vi "Transmisor SERIALvi.vi"() -> ()   [LabVIEW 2020]
uses:
  <vilib>/Instr/_visa.llb/VISA Configure Serial Port (Instr).vi
panel:
  in  "ConfigSerial":T1={"baud rate (9600)"=9600, "data bits (8)"=8, "parity (0:none)"=enum."None", "stop bits (10: 1 bit)"=10, "flow control (0:none)"=0, "VISA resource name"="", "error in (no error) 2"={"status"=FALSE, "code"=0, "source"=""}} {"flow control (0:none)" items=["None", "XON/XOFF", "RTS/CTS", "XON/XOFF & RTS/CTS", "DTR/DSR", "XON/XOFF & DTR/DSR"]; "stop bits (10: 1 bit)" items=["1.0"=10, "1.5"=15, "2.0"=20]; "data bits (8)" min=5 max=8 step=1}
  in  "Stop":bool
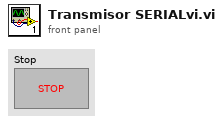
[diagram p1: front panel]
types:
  T1 = cluster{"baud rate (9600)":u32, "data bits (8)":u16, "parity (0:none)":enum16{"None", "Odd", "Even", "Mark", "Space"}, "stop bits (10: 1 bit)":u16, "flow control (0:none)":u16, "VISA resource name":refnum<visa-resource-name>, "error in (no error) 2":errorcluster}
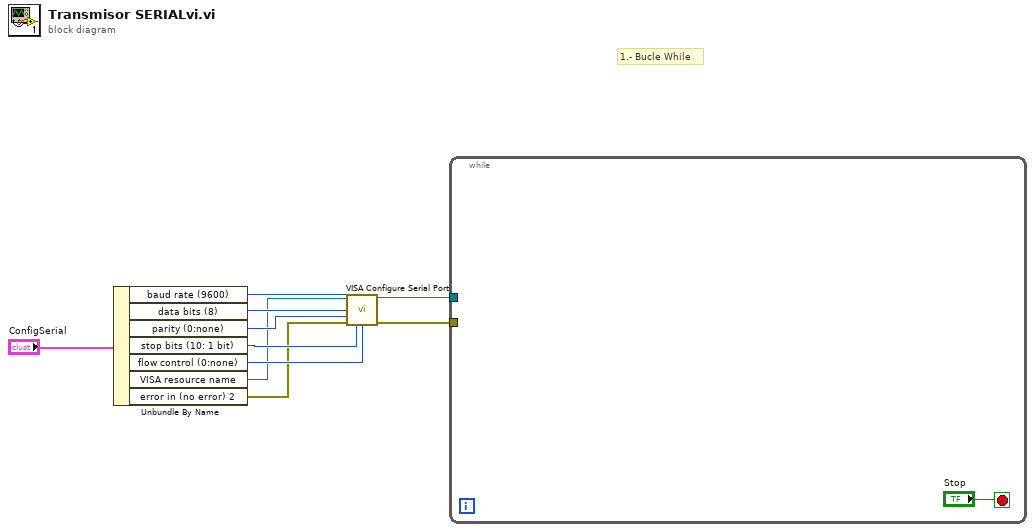
[diagram p0: block diagram]
diagram:
  # "1.- Bucle While"
  n1 = Unbundle By Name("ConfigSerial") -> ("baud rate (9600)"=w9:u32, "data bits (8)"=w8:u16, "parity (0:none)"=w7:enum16{"None", "Odd", "Even", "Mark", "Space"}, "stop bits (10: 1 bit)"=w6:u16, "flow control (0:none)"=w5:u16, "VISA resource name"=w4:refnum<visa-resource-name>, "error in (no error) 2"=w3:errorcluster)
  n2 = call-poly "VISA Configure Serial Port"("VISA resource name"=w4, "baud rate (9600)"=w9, "data bits (8)"=w8, "parity (0:none)"=w7, "error in (no error)"=w3, "stop bits (10: 1 bit)"=w6, "flow control (0:none)"=w5) -> ("VISA resource name out"=w2:refnum<visa-resource-name>, "error out"=w1:errorcluster)  [unwired: 7 in]
  n3 = while {
    tunnel: w2 -> [_]
    tunnel: w1 -> [_]
    stop <- "Stop" stop-if-true
  }
